vi "Predictive Filter Age Out.vi"(9 "Index":i32, 10 "Predictive Filter Cluster in":T1={"Previous Position "=[], "Filter Factor a"=[0.25, 0.25, 0.2], "Velocity Previous"=[], "Filter Factor ß"=[0.1, 0.1, 0.1], "Age by tag"=[]}) -> (1 "Process":bool, 2 "Predictive Filter Cluster out":T1={"Previous Position "=[], "Filter Factor a"=[0.25, 0.25, 0.2], "Velocity Previous"=[], "Filter Factor ß"=[0.1, 0.1, 0.1], "Age by tag"=[]})   [LabVIEW 2025]
uses:
  Predictive Filter Cluster.ctl
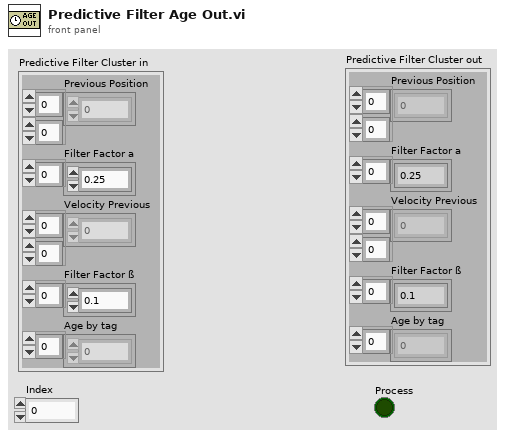
[diagram p1: front panel]
types:
  T1 = typedef "Predictive Filter Cluster.ctl" = cluster{"Previous Position ":dbl[][], "Filter Factor a":dbl[], "Velocity Previous":dbl[][], "Filter Factor ß":dbl[], "Age by tag":u32[]}
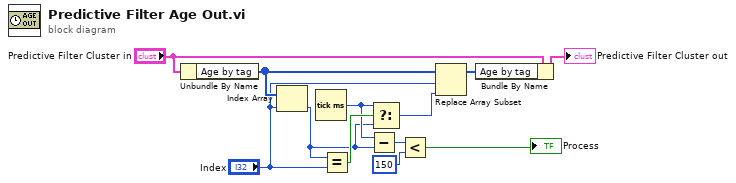
[diagram p0: block diagram]
diagram:
  n1 = Unbundle By Name("Predictive Filter Cluster in") -> ("Age by tag"=w4:u32[])
  n2 = Index Array(array=w4, index="Index") -> (element=w1:u32)
  n3 = Tick Count (ms)() -> (millisecond timer value=w6:u32)
  n4 = Equal?(x=w1, y="Index") -> (x = y?=w7:bool)
  n5 = Subtract(x=w6, y=w1) -> (x-y=w5:u32)
  n6 = Select(t=w6, s=w7, f=w1) -> (s? t:f=w8:u32)
  n7 = Less?(x=w5, y=u32 150) -> (x < y?=→"Process":bool)
  n8 = Replace Array Subset(array=w4, new element=w8, index="Index") -> (w11:u32[])
  n9 = Bundle By Name(cluster="Predictive Filter Cluster in", "Age by tag"=w11) -> (→"Predictive Filter Cluster out":T1)
